vi "SpecPage.vi"(10 "Spec Page Interface":T1 caption="规范页接口", 11 "MetaDataObj in":refnum<class "MetaDataObj.lvclass"> caption="元数据对象输入") -> (3 "MetaDataObj out":refnum<class "MetaDataObj.lvclass"> caption="元数据对象输出")   [LabVIEW 2016]
uses:
  <resource>/dialog/NewProjectWizard/Spec Page Interface.ctl
  <resource>/dialog/NewProjectWizard/MetaDataObj/MetaDataObj.lvclass
  <resource>/dialog/NewProjectWizard/MetaDataObj/MetaDataObj.lvclass/MetaDataObj.ctl
  <resource>/dialog/NewProjectWizard/MetaDataObj/Accessors/Read Overlay Pixmap.vi
  <resource>/dialog/NewProjectWizard/MetaDataObj/Accessors/Write Overlay Pixmap.vi
  <resource>/dialog/NewProjectWizard/MetaDataObj/Accessors/Write File Prefix.vi
  <resource>/dialog/NewProjectWizard/MetaDataObj/Accessors/Write Project Name.vi
  <resource>/dialog/NewProjectWizard/MetaDataObj/Accessors/Write Project Root.vi
  <resource>/dialog/NewProjectWizard/MetaDataObj/Accessors/Read Hide Prefix.vi
  <resource>/dialog/NewProjectWizard/MetaDataObj/Accessors/Read Hide Icon Overlay.vi
  <vilib>/LabVIEW Icon API/lv_icon/Classes/Icon/Icon.lvclass
  <resource>/dialog/NewProjectWizard/Icon Overlay/NI_NPW_Icon Overlay.lvlib
  <vilib>/LabVIEW Icon API/LabVIEW Icon API.lvlib
panel:
  in  "Project Name":string caption="项目名称"
  in  "Project Root":path caption="项目根目录"
  in  "File Name Prefix (Optional)":string caption="文件名称前缀（可选）"
  out "Modified Icon":picture caption="已修改图标"
  in  "Sample Icon":picture caption="样例图标"
  out "Overlay (picture)":picture caption="图层（图片）"
  in  "Edit Icon Overlay":bool caption="编辑图标图层"
  # "修改VI图标"
  # "+"
  # "="
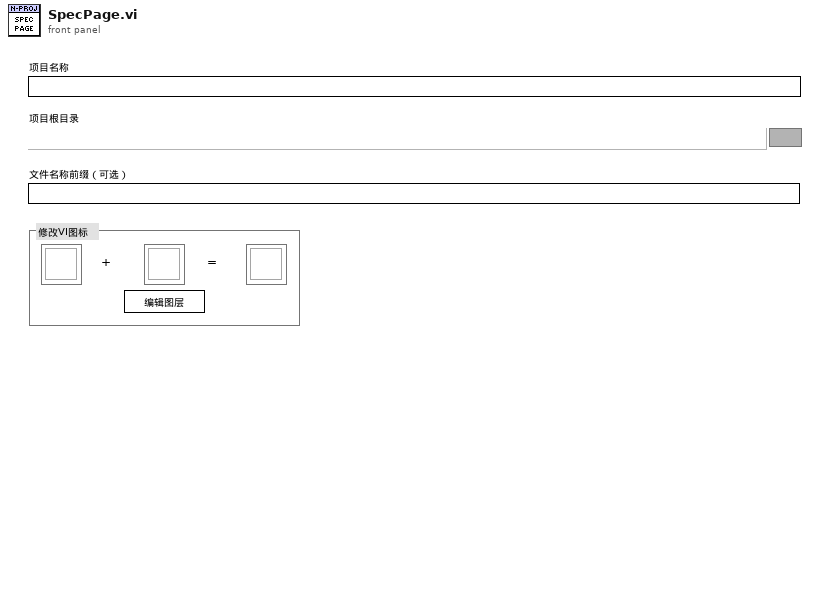
[diagram p1: front panel]
types:
  T1 = typedef "Spec Page Interface.ctl" = cluster{"\"Tab Forward To\" Refnum":refnum<vi>, "\"Tab Backward To\" Refnum":refnum<vi>, "Errors":refnum<user-event>, "Quit":refnum<user-event>}
  T2 = typedef "imagedata.ctl" = cluster{"image type":i32, "image depth":i32, "image":u8[], "mask":u8[], "colors":u32[], "Rectangle":cluster{"left":i16, "top":i16, "right":i16, "bottom":i16}}
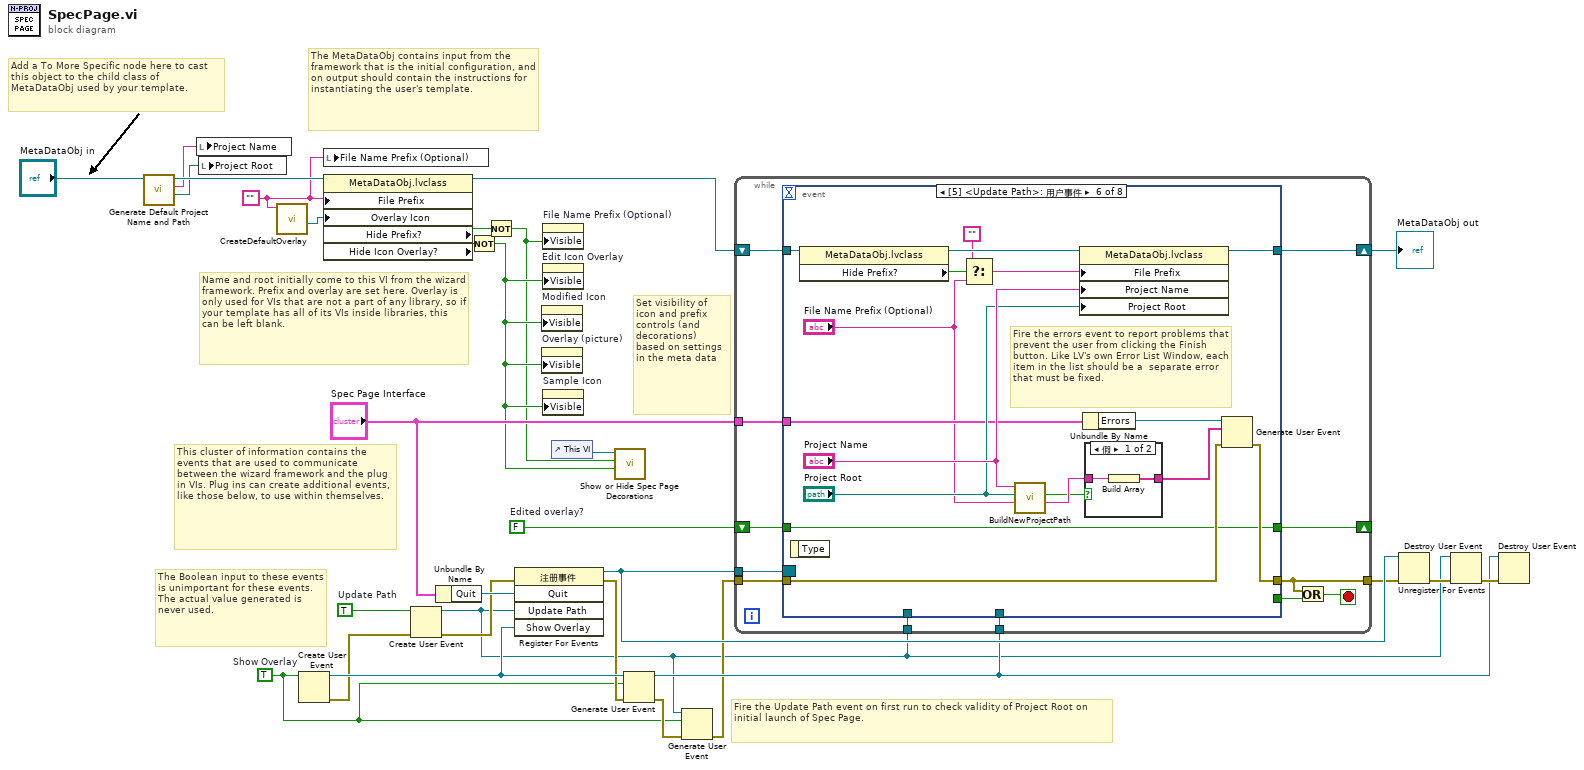
[diagram p0: block diagram]
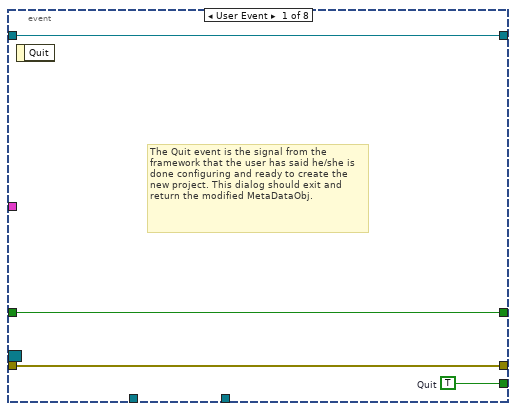
[diagram p2: hidden frame]
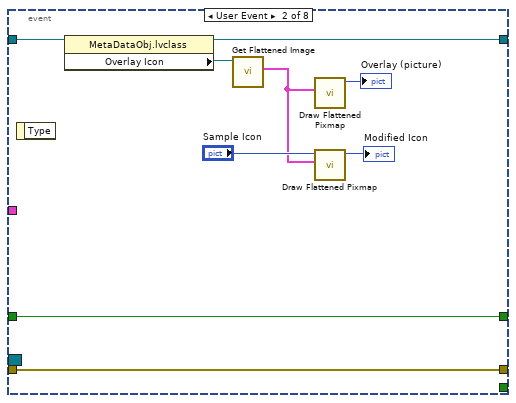
[diagram p3: hidden frame]
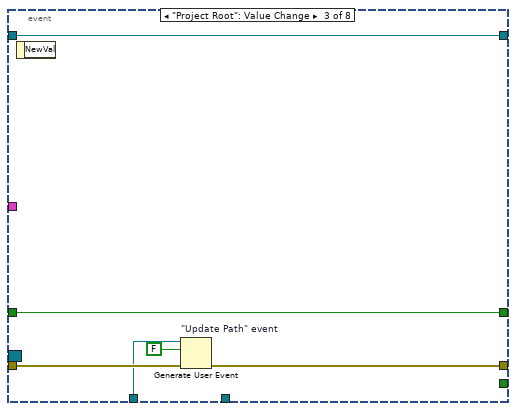
[diagram p4: hidden frame]
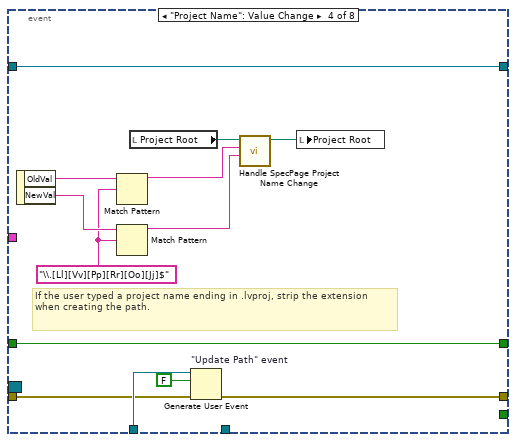
[diagram p5: hidden frame]
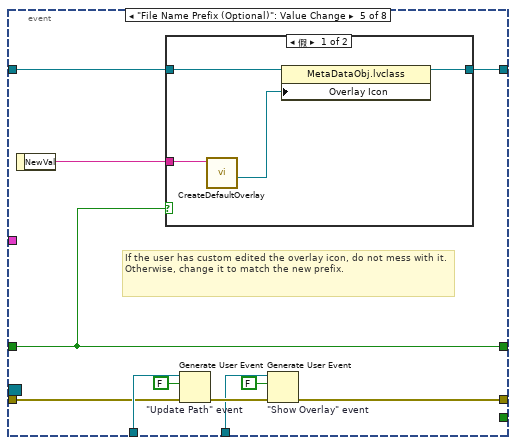
[diagram p6: hidden frame]
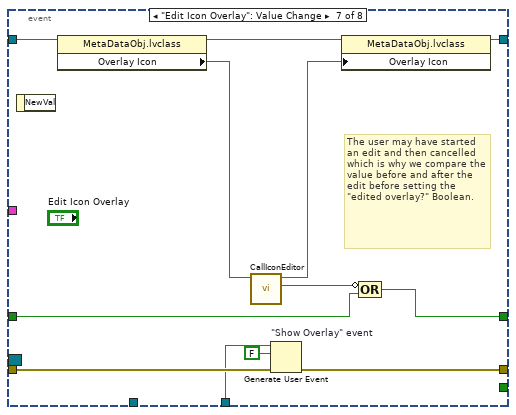
[diagram p9: hidden frame]
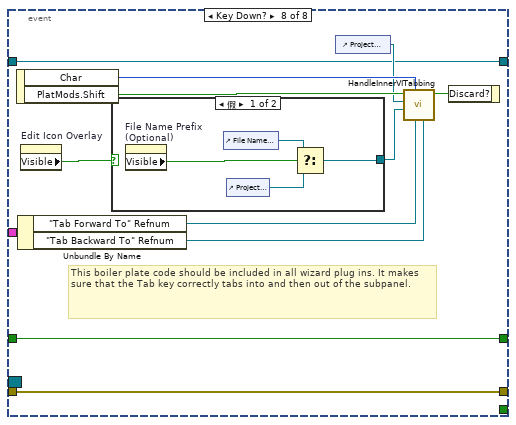
[diagram p10: hidden frame]
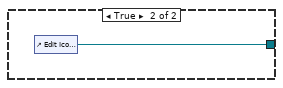
[diagram p11: hidden frame]
diagram:
  w1 = ""
  w21 = FALSE  # Edited overlay?
  w14 = TRUE  # Show Overlay
  w26 = TRUE  # Update Path
  # "Set visibility of icon and prefix controls (and decorations) based on settings in the meta data"
  # "Fire the Update Path event on first run to check validity of Project Root on initial launch of Spec Page."
  # "The Boolean input to these events is unimportant for these events. The actual value generated is never used."
  # "This cluster of information contains the events that are used to communicate between the wizard framework and the plug in VIs. Plug ins can create additional events, like those below, to use within themselves."
  # "The MetaDataObj contains input from the framework that is the initial configuration, and on output should contain the instructions for instantiating the user's template."
  # "Add a To More Specific node here to cast this object to the child class of MetaDataObj used by your template."
  # "Name and root initially come to this VI from the wizard framework. Prefix and overlay are set here. Overlay is only used for VIs that are not a part of any library, so if your template has all of its VIs inside libraries, this can be left blank."
  n1 = call <resource>:"Generate Default Project Name and Path.vi"("DNL_MetaDataObj in"="MetaDataObj in") -> ("Project Root"=w2:path, "Project Name"=w3:string, "DNL_MetaDataObj out"=w4:refnum<class "MetaDataObj.lvclass">)  [unwired: 8 in]
  n2 = local write "Project Name"(w3) -> ()
  n3 = local write "Project Root"(w2) -> ()
  n4 = call <resource>:"CreateDefaultOverlay.vi"("File Prefix"=w1) -> ("Overlay Icon"=w12:refnum<class "Icon.lvclass">)  [unwired: 8 in, 2 out]
  n5 = Create User Event(user event datatype=w14) -> (user event=w20:refnum<user-event>, error out=w17:errorcluster)  [unwired: 1 in]
  n6 = local write "File Name Prefix (Optional)"(w1) -> ()
  n7 = property class="MetaDataObj.lvclass"(reference=w4, "File Prefix"=w1, "Overlay Icon"=w12) -> (reference out=w11:refnum<class "MetaDataObj.lvclass">, "Hide Prefix?"=w10:bool, "Hide Icon Overlay?"=w9:bool)  [unwired: 1 in, 1 out]
  n8 = Create User Event(user event datatype=w26, error in=w17) -> (user event=w13:refnum<user-event>, error out=w25:errorcluster)
  n9 = Unbundle By Name("Spec Page Interface") -> ("Quit"=w30:refnum<user-event>)
  n10 = Not(x=w9) -> (.not. x?=w7:bool)
  n11 = Not(x=w10) -> (.not. x?=w6:bool)
  n12 = register-events(error in=w25, w30, w13, w20) -> (reference out=w29:refnum<event-registration>, error out=w18:errorcluster)  [unwired: 1 in]
  n13 = property on="Modified Icon" class="Pict"("Visible"=w7) -> ()  [unwired: 2 in, 2 out]
  n14 = property on="Overlay (picture)" class="Pict"("Visible"=w7) -> ()  [unwired: 2 in, 2 out]
  n15 = property on="File Name Prefix (Optional)" class="Str"("Visible"=w6) -> ()  [unwired: 2 in, 2 out]
  n16 = property on="Edit Icon Overlay" class="Bool"("Visible"=w7) -> ()  [unwired: 2 in, 2 out]
  n17 = property on="Sample Icon" class="Pict"("Visible"=w7) -> ()  [unwired: 2 in, 2 out]
  n18 = control-ref of="This VI"() -> (w8:refnum<vi>)
  n19 = call <resource>:"Show or Hide Spec Page Decorations.vi"("Icon Visible"=w7, "Prefix Visible"=w6, "Spec Page refnum"=w8) -> ()  [unwired: 9 in]
  n20 = Generate User Event(user event=w20, event data cluster=w14, error in=w18) -> (user event out=w19:refnum<user-event>, error out=w16:errorcluster)  [unwired: 1 in]
  n21 = Generate User Event ("\"Update Path\" event")(user event=w13, event data cluster=w14, error in=w16) -> (error out=w15:errorcluster)  [unwired: 1 in, 1 out]
  n22 = while {
    tunnel: "Spec Page Interface" -> [w40]
    shift-right: [w39] -> w23
    shift-left: w11 -> [w38]
    tunnel: w29 -> [w42]
    tunnel: w15 -> [w41]
    tunnel: [w35] -> w27
    tunnel: w13 -> [w34]
    tunnel: w19 -> [w33]
    shift-right: [w31] -> _
    shift-left: w21 -> [w32]
    stop <- w37 stop-if-true
    n23 = event shown="[5] <Update Path>: 用户事件" {
      selector: w42 -> [_ _ _ _ _ _ _ _]
      dyn-events: _ -> [_ _ _ _ _ _ _ _]
      timeout: _ -> [_ _ _ _ _ _ _ _]
      tunnel: w40 -> [_ _ _ _ _ w101 _ w129]
      tunnel: [w46 _ _ _ _ _ _ _] -> w36
      tunnel: [w45 w55 w59 w70 w77 w99 w116 w126] -> w35
      tunnel: w41 -> [w45 w55 w60 w71 w83 w100 w117 w126]
      tunnel: [w44 w50 w61 w67 w80 w97 w121 w125] -> w39
      tunnel: w38 -> [w44 w51 w61 w67 w81 w98 w120 w125]
      tunnel: w34 -> [_ _ w58 w72 w85 _ _ _]
      tunnel: w33 -> [_ _ _ _ w76 _ w115 _]
      tunnel: w32 -> [w43 w49 w56 w68 w75 w96 w114 w124]
      tunnel: [w43 w49 w56 w68 w75 w96 w113 w124] -> w31
      event User Event {
        w46 = TRUE  # Quit
        # "The Quit event is the signal from the framework that the user has said he/she is done configuring and ready to create the new project. This dialog should exit and return the modified MetaDataObj."
        n24 = event-data() -> ()  [unwired: 1 in, 1 out]
      }
      event User Event {
        n25 = event-data() -> ()  [unwired: 1 in, 1 out]
        n26 = property class="MetaDataObj.lvclass"(reference=w51) -> (reference out=w50:refnum<class "MetaDataObj.lvclass">, "Overlay Icon"=w48:refnum<class "Icon.lvclass">)  [unwired: 1 in, 1 out]
        n27 = call <vilib>:"Get Flattened Image.vi"("lv_icon.lvlib:Icon.lvclass in"=w48) -> ("Color Image"=w47:T2)  [unwired: 7 in, 3 out]
        n28 = call <vilib>:"Draw Flattened Pixmap.vi"("image data"=w47) -> ("new picture"=→"Overlay (picture)":picture)  [unwired: 8 in]
        n29 = call <vilib>:"Draw Flattened Pixmap.vi"("image data"=w47, "picture"="Sample Icon") -> ("new picture"=→"Modified Icon":picture)  [unwired: 7 in]
      }
      event "Project Root": Value Change {
        n30 = event-data() -> ()  [unwired: 1 in, 1 out]
        n31 = Generate User Event "\"Update Path\" event"(user event=w58, event data cluster=FALSE ("event data"), error in=w60) -> (error out=w59:errorcluster)  [unwired: 1 in, 1 out]
      }
      event "Project Name": Value Change {
        w62 = "\\.[Ll][Vv][Pp][Rr][Oo][Jj]$" ("regular expression")
        # "If the user typed a project name ending in .lvproj, strip the extension when creating the path."
        n32 = event-data() -> ("OldVal"=w64:string, "NewVal"=w66:string)  [unwired: 1 in]
        n33 = Match Pattern(string=w64, regular expression=w62) -> (before substring=w63:string)  [unwired: 1 in, 3 out]
        n34 = Match Pattern(string=w66, regular expression=w62) -> (before substring=w65:string)  [unwired: 1 in, 3 out]
        n35 = local read "Project Root"() -> (w74:path)
        n36 = Generate User Event "\"Update Path\" event"(user event=w72, event data cluster=FALSE ("event data"), error in=w71) -> (error out=w70:errorcluster)  [unwired: 1 in, 1 out]
        n37 = call <resource>:"Handle SpecPage Project Name Change.vi"("Project Name New Value"=w65, "Project Name Old Value"=w63, "Project Root in"=w74) -> ("Project Root out"=w73:path)  [unwired: 8 in]
        n38 = local write "Project Root"(w73) -> ()
      }
      event "File Name Prefix (Optional)": Value Change {
        # "If the user has custom edited the overlay icon, do not mess with it. Otherwise, change it to match the new prefix."
        n39 = event-data() -> ("NewVal"=w82:string)  [unwired: 1 in]
        n40 = case shown="假" w75 {
          tunnel: w82 -> [w89 _]
          tunnel: w81 -> [w88 w90]
          tunnel: [w87 w90] -> w80
          frame False {
            n41 = call <resource>:"CreateDefaultOverlay.vi"("File Prefix"=w89) -> ("Overlay Icon"=w86:refnum<class "Icon.lvclass">)  [unwired: 8 in, 2 out]
            n42 = property class="MetaDataObj.lvclass"(reference=w88, "Overlay Icon"=w86) -> (reference out=w87:refnum<class "MetaDataObj.lvclass">)  [unwired: 1 in, 1 out]
          }
          frame True {
          }
        }
        n43 = Generate User Event "\"Update Path\" event"(user event=w85, event data cluster=FALSE ("event data"), error in=w83) -> (error out=w78:errorcluster)  [unwired: 1 in, 1 out]
        n44 = Generate User Event "\"Show Overlay\" event"(user event=w76, event data cluster=FALSE ("event data"), error in=w78) -> (error out=w77:errorcluster)  [unwired: 1 in, 1 out]
      }
      event User Event {
        # "Fire the errors event to report problems that prevent the user from clicking the Finish button. Like LV's own Error List Window, each item in the list should be a  separate error that must be fixed."
        n45 = event-data() -> ()  [unwired: 1 in, 1 out]
        n46 = property class="MetaDataObj.lvclass"(reference=w98) -> (reference out=w95:refnum<class "MetaDataObj.lvclass">, "Hide Prefix?"=w93:bool)  [unwired: 1 in, 1 out]
        n47 = Select(t="", s=w93, f="File Name Prefix (Optional)") -> (s? t:f=w92:string)
        n48 = call <resource>:"BuildNewProjectPath.vi"("File Prefix"="File Name Prefix (Optional)", "Project Root"="Project Root", "Project Name"="Project Name") -> ("Error Message"=w104:string, "Valid?"=w102:bool)  [unwired: 6 in, 1 out]
        n49 = property class="MetaDataObj.lvclass"(reference=w95, "File Prefix"=w92, "Project Name"="Project Name", "Project Root"="Project Root") -> (reference out=w97:refnum<class "MetaDataObj.lvclass">)  [unwired: 1 in, 1 out]
        n50 = Unbundle By Name(w101) -> ("Errors"=w107:refnum<user-event>)
        n51 = case shown="假" w102 {
          tunnel: w104 -> [w109 _]
          tunnel: [w108 _] -> w103
          frame False {
            n52 = Build Array(w109) -> (w108:string[])
          }
          frame True {
          }
        }
        n53 = Generate User Event(user event=w107, event data cluster=w103, error in=w100) -> (error out=w99:errorcluster)  [unwired: 1 in, 1 out]
      }
      event "Edit Icon Overlay": Value Change {
        # "The user may have started an edit and then cancelled which is why we compare the value before and after the edit before setting the \"edited overlay?\" Boolean."
        n54 = event-data() -> ()  [unwired: 1 in, 1 out]
        n55 = property class="MetaDataObj.lvclass"(reference=w120) -> (reference out=w119:refnum<class "MetaDataObj.lvclass">, "Overlay Icon"=w112:refnum<class "Icon.lvclass">)  [unwired: 1 in, 1 out]
        n56 = call <resource>:"CallIconEditor.vi"("Icon in"=w112) -> ("Canceled?"=w110:bool, "Icon out"=w111:refnum<class "Icon.lvclass">)  [unwired: 9 in]
        n57 = Generate User Event "\"Show Overlay\" event"(user event=w115, event data cluster=FALSE ("event data"), error in=w117) -> (error out=w116:errorcluster)  [unwired: 1 in, 1 out]
        n58 = property class="MetaDataObj.lvclass"(reference=w119, "Overlay Icon"=w111) -> (reference out=w121:refnum<class "MetaDataObj.lvclass">)  [unwired: 1 in, 1 out]
        n59 = Compound Arithmetic op=OR(invert w110, w114) -> (w113:bool)
      }
      event Key Down? {
        # "This boiler plate code should be included in all wizard plug ins. It makes sure that the Tab key correctly tabs into and then out of the subpanel."
        n60 = event-data() -> ("Char"=w132:i16, "PlatMods.Shift"=w131:bool)  [unwired: 1 in]
        n61 = Unbundle By Name(w129) -> ("\"Tab Forward To\" Refnum"=w128:refnum<vi>, "\"Tab Backward To\" Refnum"=w127:refnum<vi>)
        n62 = property on="Edit Icon Overlay" class="Bool"() -> ("Visible"=w123:bool)  [unwired: 2 in, 2 out]
        n63 = case shown="假" w123 {
          tunnel: [w134 w138] -> w122
          frame False {
            n64 = property on="File Name Prefix (Optional)" class="Str"() -> ("Visible"=w137:bool)  [unwired: 2 in, 2 out]
            n65 = control-ref of="File Name Prefix (Optional)"() -> (w136:refnum<vi>)
            n66 = control-ref of="Project Root"() -> (w135:refnum<vi>)
            n67 = Select(t=w136, s=w137, f=w135) -> (s? t:f=w134:refnum<vi>)
          }
          frame True {
            n68 = control-ref of="Edit Icon Overlay"() -> (w138:refnum<vi>)
          }
        }
        n69 = control-ref of="Project Name"() -> (w130:refnum<vi>)
        n70 = call <resource>:"HandleInnerVITabbing.vi"("Tab Backward To"=w127, "Tab Forward To"=w128, "Char"=w132, "Last Control"=w122, "First Control"=w130, "Shift"=w131) -> ("Discard"=w133:bool)  [unwired: 5 in]
        n71 = event-data("Discard?"=w133) -> ()  [unwired: 1 in, 1 out]
      }
    }
    n72 = Or(x=w35, y=w36) -> (x .or. y?=w37:bool)
  }
  "MetaDataObj out" <- w23
  n73 = Unregister For Events(event registration refnum=w29, error in=w27) -> (error out=w24:errorcluster)
  n74 = Destroy User Event(user event=w13, error in=w24) -> (error out=w22:errorcluster)
  n75 = Destroy User Event(user event=w19, error in=w22) -> ()  [unwired: 1 out]
